vi "GetTime Stamp.vi"(7 "key description":string, 8 "sections":string[](array[string]), 9 "time stamp":timestamp, 11 "info data":string) -> (0 "sections out":string[](array[string]), 2 "value":timestamp, 3 "info data out":string)   [LabVIEW 2013, in "infolib.lvlib"]
doc: "Add a new numeric key to Info Data string. If section exists in Info Data string, inserts key into this section."
uses:
  infolib.lvlib
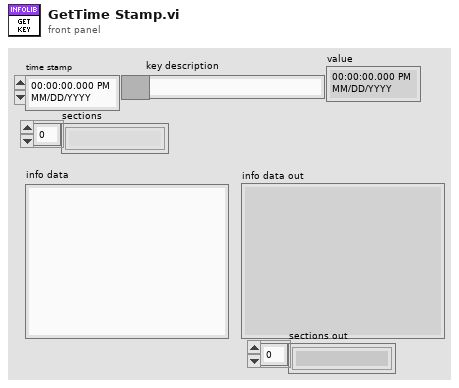
[diagram p1: front panel]
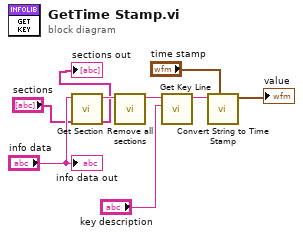
[diagram p0: block diagram]
diagram:
  n1 = call "Get Section.vi"("sections"="sections", "info data"="info data") -> ("sections out"=→"sections out":string[], "section part"=w9:string)  [unwired: 7 in, 1 out]
  n2 = call "Remove all sections.vi"("info data"=w9) -> ("info data out"=w8:string)  [unwired: 10 in]
  n3 = call "Get Key Line.vi"("key description"="key description", "info data"=w8) -> ("key value"=w4:string)  [unwired: 9 in]
  n4 = call "Convert String to Time Stamp.vi"("default value of time stamp"="time stamp", "string"=w4) -> ("time stamp out"=→"value":timestamp)  [unwired: 9 in]
  "info data out" <- "info data"
